vi "test_CCDSetAndGetTimerResolution.vi"(7 "Test should pass":bool=TRUE, 8 "error in":errorcluster, 9 "tear down connection":bool=TRUE, 10 "set-up a connection":bool=TRUE, 11 "device selection":enum16{"monochromator", "CCD", "SCD"}(ring)=enum."CCD") -> (0 "error out":errorcluster)   [LabVIEW 2023]
uses:
  Source/Classes/Mono/Monochromator.lvclass
  Source/Classes/CCD/CCD.lvclass
  Source/Classes/SCD/SCD.lvclass
  Source/Classes/CCD/GainTokenEnum.ctl
  <vilib>/addons/_JKI Toolkits/Caraya/classes/Assert/Assert Equal Value and Type_Variant.vi
  <vilib>/addons/_JKI Toolkits/Caraya/classes/Assert/Assert Not Error.vi
  Source/Classes/GenericDevice/GenericDevice.lvclass
  <vilib>/addons/_JKI Toolkits/Caraya/classes/Test/Test.lvclass
  <vilib>/addons/_JKI Toolkits/Caraya/classes/Assert/Assert.lvclass
  Source/Classes/CCD/TimerResolutionEnum.ctl
panel:
  # "Connector Pane"
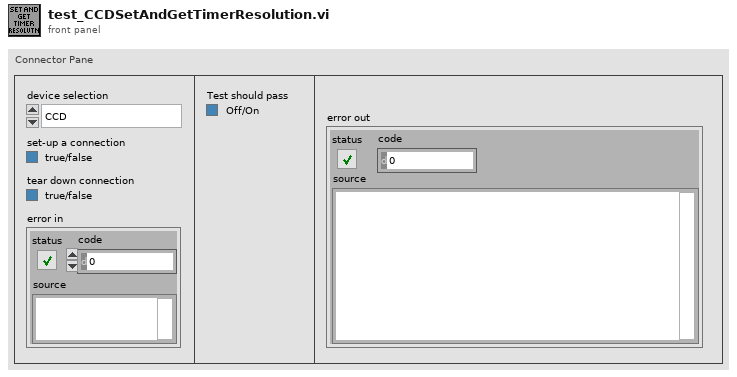
[diagram p1: front panel]
types:
  T1 = typedef "CCD.lvclass/TimerResolutionEnum.ctl" = enum16{"0 - Sets the timer resolution to 1000 microseconds", "1 - Sets the timer resolution to 1 microsecond"}
  T2 = typedef "CCD.lvclass/GainTokenEnum.ctl" = enum16{"High Light", "Best Dynamic Range", "High Sensitivity"}
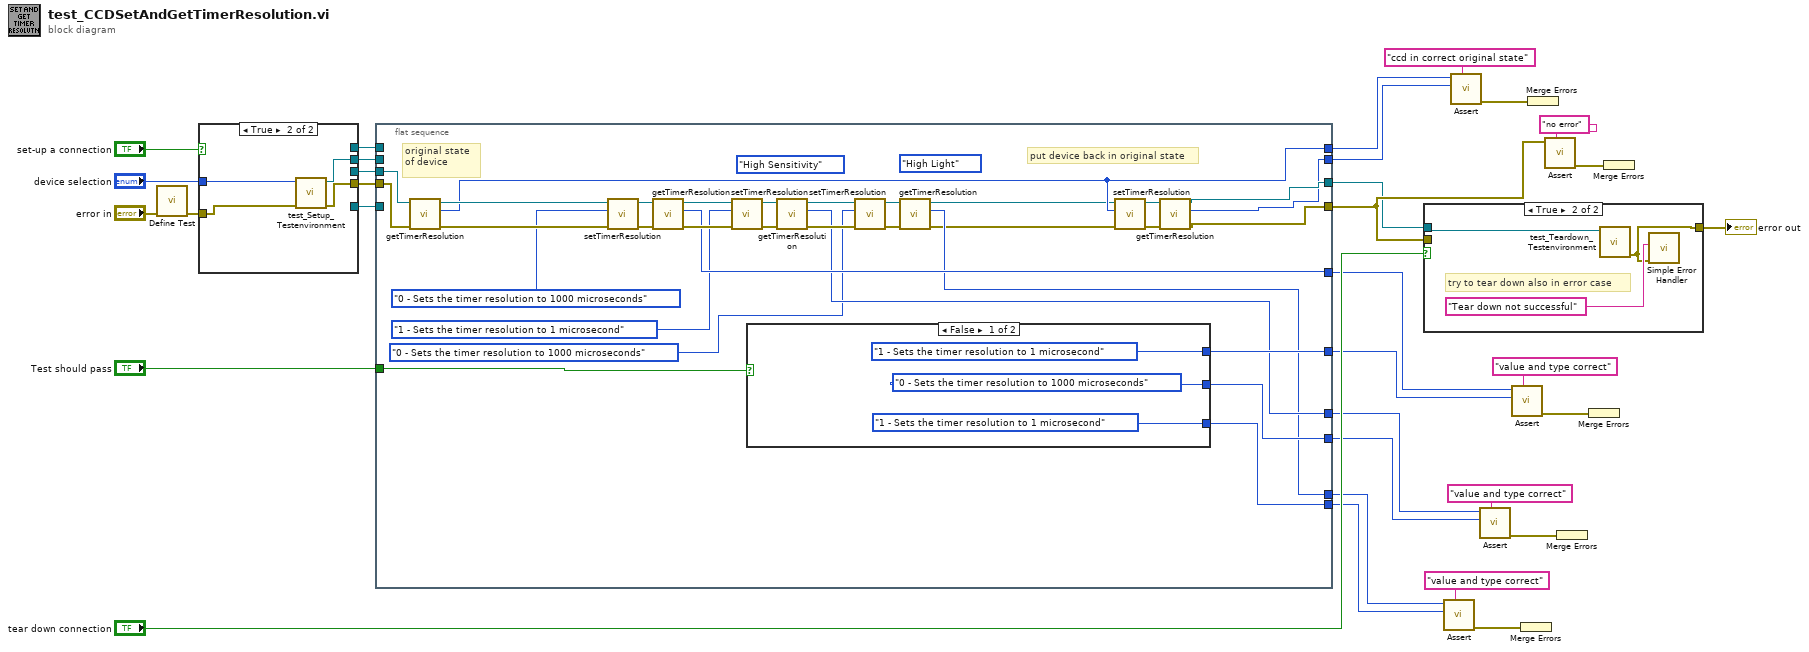
[diagram p0: block diagram]
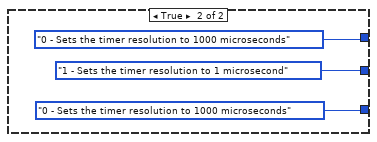
[diagram p2: hidden frame]
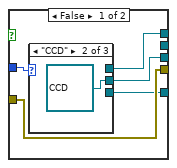
[diagram p3: hidden frame]
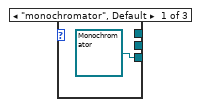
[diagram p4: hidden frame]
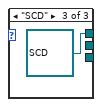
[diagram p5: hidden frame]
diagram:
  n1 = call <vilib>:"Define Test.vi"("error in (no error)"="error in") -> ("error out"=w28:errorcluster)  [unwired: 9 in, 1 out]
  n2 = case shown="True" "set-up a connection" {
    tunnel: w28 -> [w37 w44]
    tunnel: [w37 w43] -> w30
    tunnel: "device selection" -> [w36 w42]
    tunnel: [_ w41] -> w27
    tunnel: [w35 _] -> w26
    tunnel: [w34 _] -> w25
    tunnel: [w33 _] -> w24
    frame False {
      n3 = case shown="\"CCD\"" w36 {
        tunnel: [refnum<class "Monochromator.lvclass"> refnum ("Monochromator.lvclass") _ _] -> w35
        tunnel: [_ refnum<class "CCD.lvclass"> refnum ("CCD in") _] -> w34
        tunnel: [_ _ refnum<class "SCD.lvclass"> refnum ("SCD.lvclass")] -> w33
        frame "monochromator", Default {
        }
        frame "CCD" {
        }
        frame "SCD" {
        }
      }
    }
    frame True {
      n4 = call "test_Setup_Testenvironment.vi"("error in"=w44, "device selection"=w42) -> ("error out"=w43:errorcluster, "GenericDevice.lvclass"=w41:refnum<class "GenericDevice.lvclass">)  [unwired: 7 in, 1 out]
    }
  }
  n5 = flat-sequence {
    tunnel: w30 -> [w74]
    tunnel: w27 -> [_]
    tunnel: w26 -> [_]
    tunnel: w25 -> [w75]
    tunnel: w24 -> [_]
    tunnel: [w58] -> w19
    tunnel: "Test should pass" -> [w76]
    tunnel: [w57] -> w18
    tunnel: [w56] -> w15
    tunnel: [w59] -> w14
    tunnel: [w55] -> w13
    tunnel: [w53] -> w11
    tunnel: [w50] -> w9
    tunnel: [w54] -> w12
    tunnel: [w52] -> w10
    tunnel: [w51] -> w8
    frame #0 {
      (unwired) GainTokenEnum."High Light" ("gain token (enum)")
      (unwired) GainTokenEnum."High Sensitivity" ("gain token (enum)")
      # "put device back in original state"
      # "original state of device"
      n6 = call "getTimerResolution.vi"("error in (no error)"=w74, "CCD in"=w75) -> ("error out"=w60:errorcluster, "resolution"=w59:T1, "CCD out"=w61:refnum<class "CCD.lvclass">)  [unwired: 7 in]
      n7 = call "setTimerResolution.vi"("error in (no error)"=w60, "resolution"=TimerResolutionEnum."0 - Sets the timer resolution to 1000 microseconds", "CCD in"=w61) -> ("error out"=w65:errorcluster, "CCD out"=w64:refnum<class "CCD.lvclass">)  [unwired: 5 in, 2 out]
      n8 = call "getTimerResolution.vi"("error in (no error)"=w65, "CCD in"=w64) -> ("error out"=w69:errorcluster, "resolution"=w55:T1, "CCD out"=w68:refnum<class "CCD.lvclass">)  [unwired: 7 in]
      n9 = call "setTimerResolution.vi"("error in (no error)"=w69, "resolution"=TimerResolutionEnum."1 - Sets the timer resolution to 1 microsecond", "CCD in"=w68) -> ("error out"=w66:errorcluster, "CCD out"=w67:refnum<class "CCD.lvclass">)  [unwired: 5 in, 2 out]
      n10 = case shown="False" w76 {
        tunnel: [TimerResolutionEnum."1 - Sets the timer resolution to 1 microsecond" ("resolution") TimerResolutionEnum."0 - Sets the timer resolution to 1000 microseconds" ("resolution")] -> w54
        tunnel: [TimerResolutionEnum."0 - Sets the timer resolution to 1000 microseconds" ("resolution") TimerResolutionEnum."1 - Sets the timer resolution to 1 microsecond" ("resolution")] -> w52
        tunnel: [TimerResolutionEnum."1 - Sets the timer resolution to 1 microsecond" ("resolution") TimerResolutionEnum."0 - Sets the timer resolution to 1000 microseconds" ("resolution")] -> w51
        frame False {
        }
        frame True {
        }
      }
      n11 = call "getTimerResolution.vi"("error in (no error)"=w66, "CCD in"=w67) -> ("error out"=w71:errorcluster, "resolution"=w53:T1, "CCD out"=w70:refnum<class "CCD.lvclass">)  [unwired: 7 in]
      n12 = call "setTimerResolution.vi"("error in (no error)"=w71, "resolution"=TimerResolutionEnum."0 - Sets the timer resolution to 1000 microseconds", "CCD in"=w70) -> ("error out"=w63:errorcluster, "CCD out"=w62:refnum<class "CCD.lvclass">)  [unwired: 5 in, 2 out]
      n13 = call "getTimerResolution.vi"("error in (no error)"=w63, "CCD in"=w62) -> ("error out"=w45:errorcluster, "resolution"=w50:T1, "CCD out"=w46:refnum<class "CCD.lvclass">)  [unwired: 7 in]
      n14 = call "setTimerResolution.vi"("error in (no error)"=w45, "resolution"=w59, "CCD in"=w46) -> ("error out"=w72:errorcluster, "CCD out"=w73:refnum<class "CCD.lvclass">)  [unwired: 5 in, 2 out]
      n15 = call "getTimerResolution.vi"("error in (no error)"=w72, "CCD in"=w73) -> ("error out"=w58:errorcluster, "resolution"=w56:T1, "CCD out"=w57:refnum<class "CCD.lvclass">)  [unwired: 7 in]
    }
  }
  n16 = case shown="True" "tear down connection" {
    tunnel: w18 -> [_ w85]
    tunnel: [w83 w84] -> w1
    tunnel: w19 -> [w83 _]
    frame False {
    }
    frame True {
      # "try to tear down also in error case"
      n17 = call "test_Teardown_Testenvironment.vi"("GenericDevice.lvclass"=w85) -> ("error out"=w84:errorcluster)  [unwired: 9 in, 1 out]
      n18 = call <vilib>:"Simple Error Handler.vi"("error source (\" \")"="Tear down not successful" ("error source (\" \")"), "error in (no error)"=w84) -> ()  [unwired: 3 in, 5 out]
    }
  }
  "error out" <- w1
  n19 = call-poly <vilib>:"Assert.vi"("Label"="value and type correct" ("Label (VI Title)"), "Y"=w8, "X"=w9) -> ("error out"=w7:errorcluster)  [unwired: 7 in, 1 out]
  n20 = call-poly <vilib>:"Assert.vi"("Label"="ccd in correct original state" ("Label (VI Title)"), "Y"=w15, "X"=w14) -> ("error out"=w17:errorcluster)  [unwired: 7 in, 1 out]
  n21 = call-poly <vilib>:"Assert.vi"("Label"="value and type correct" ("Label (VI Title)"), "Y"=w10, "X"=w11) -> ("error out"=w3:errorcluster)  [unwired: 7 in, 1 out]
  n22 = call-poly <vilib>:"Assert.vi"("Label"="value and type correct" ("Label (VI Title)"), "Y"=w12, "X"=w13) -> ("error out"=w4:errorcluster)  [unwired: 7 in, 1 out]
  n23 = Merge Errors(w7) -> ()  [unwired: 1 out]
  n24 = Merge Errors(w17) -> ()  [unwired: 1 out]
  n25 = call-poly <vilib>:"Assert.vi"("Label"="no error" ("Label (VI Title)"), "Not Error?"=w19) -> ("error out"=w21:errorcluster)  [unwired: 8 in, 1 out]
  n26 = Merge Errors(w3) -> ()  [unwired: 1 out]
  n27 = Merge Errors(w4) -> ()  [unwired: 1 out]
  n28 = Merge Errors(w21) -> ()  [unwired: 1 out]
